vi "Index.vi"(8 "error in (no error)":errorcluster, 10 "Index":i32, 11 "Cluster Array in":refnum<class "Cluster Array.lvclass">) -> (0 "error out":errorcluster, 3 "Indexed element":refnum<class "Generic Data.lvclass">)   [LabVIEW 2020, in "Data.lvlib" / "Cluster Array.lvclass"]
doc: "Index an element from 'Generic Data in'.\nThis implementation returns a generic U32 class with the indexed U32."
uses:
  Cluster Array.lvclass
  Generic Data.lvclass
  Cluster Array.lvclass/Cluster Array.ctl
  Cluster/Cluster.lvclass
  C:/Users/Henri/OneDrive/LabVIEW/Framework/Data/Generic Data/Generic Data.lvclass
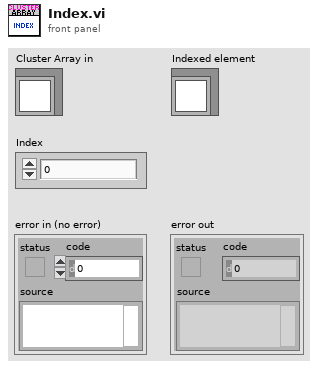
[diagram p1: front panel]
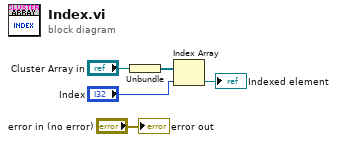
[diagram p0: block diagram]
diagram:
  n1 = Unbundle("Cluster Array in") -> (w4:refnum<class "Cluster.lvclass">[])
  n2 = Index Array(array=w4, index="Index") -> (element=→"Indexed element":refnum<class "Cluster.lvclass">)
  "error out" <- "error in (no error)"
